vi "New Waveform Data Reference.vi"(5 "Waveform Data":cluster{"t0":dbl, "dt":dbl, "y":csg[]}, 9 "error in (no error)":errorcluster) -> (6 "Waveform Data Reference":refnum<data-value>, 10 "error out":errorcluster)   [LabVIEW 2016, in "Common.lvlib"]
uses:
  Common.lvlib
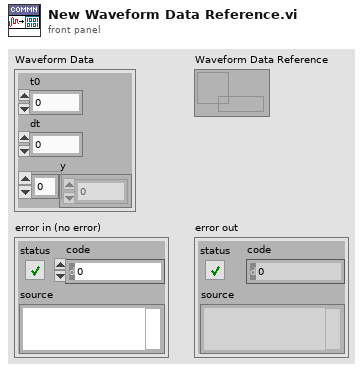
[diagram p1: front panel]
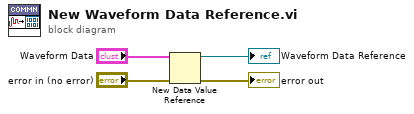
[diagram p0: block diagram]
diagram:
  n1 = New Data Value Reference(data value="Waveform Data", error in="error in (no error)") -> (data value reference=→"Waveform Data Reference":refnum<data-value>, error out=→"error out":errorcluster)
